vi "UPdataMessage.vi"(8 "错误输入（无错误）":errorcluster, 11 "Str引用句柄":refnum<vi>) -> (0 "error out":errorcluster)   [LabVIEW 2017]
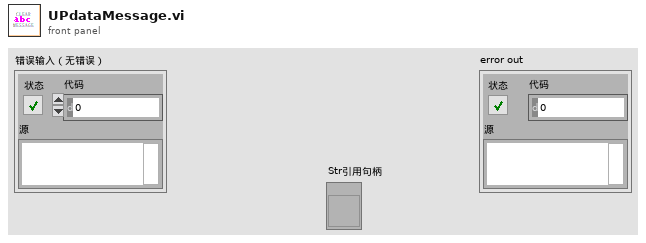
[diagram p1: front panel]
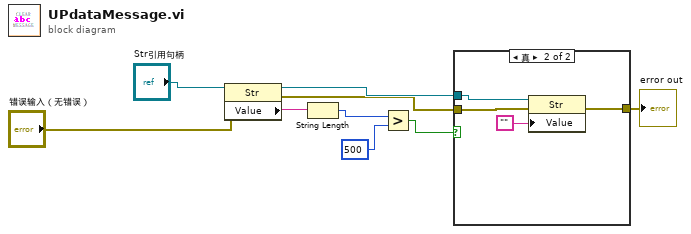
[diagram p0: block diagram]
diagram:
  n1 = property class="Str"(reference="Str引用句柄", error in="错误输入（无错误）") -> (reference out=w3:refnum<vi>, error out=w2:errorcluster, "Value"=w5:string)
  n2 = String Length(string=w5) -> (length=w7:i32)
  n3 = Greater?(x=w7, y=500) -> (0:w4:bool)
  n4 = case shown="真" w4 {
    tunnel: w3 -> [_ w14]
    tunnel: w2 -> [w10 w13]
    tunnel: [w10 w12] -> w1
    frame False {
    }
    frame True {
      n5 = property class="Str"(reference=w14, error in=w13, "Value"="") -> (error out=w12:errorcluster)  [unwired: 1 out]
    }
  }
  "error out" <- w1
